vi "Get Computer Resources.vi"(8 "error in (no error)":errorcluster) -> (0 "error out":errorcluster, 3 "Computer Resources":T1)   [LabVIEW 2020]
doc: "This VI collects via the system data API the available computing resources."
uses:
  Type Definitions/Computer Resources.ctl
  Type Definitions/Payload Class.ctl
  Type Definitions/Enum - Metadata.ctl
  <resource>/objmgr/nicontrollersysapi.rc
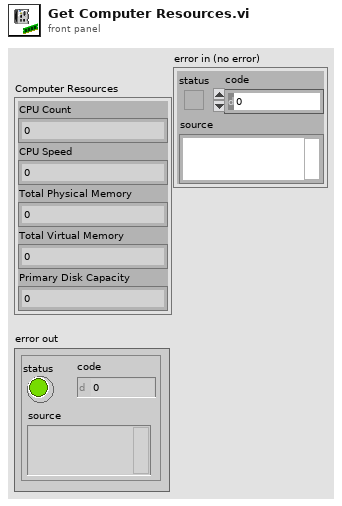
[diagram p1: front panel]
types:
  T1 = typedef "Computer Resources.ctl" = cluster{"CPU Count":i32, "CPU Speed":u32, "Total Physical Memory":dbl, "Total Virtual Memory":dbl, "Primary Disk Capacity":dbl}
  T2 = typedef "Enum - Metadata.ctl" = enum16{"Computer Metadata", "Computer Resources", "RT Image Metadata", "Startup Settings", "Telemetry Recorder Status"}
  T3 = typedef "Payload Class.ctl" = enum16{"System State", "Parameters", "Metadata", "Software Monitor", "Data", "Commands"}
  T4 = typedef "System Resources.ctl" = cluster{"System Session":refnum<k21>, "System Resource":refnum<k20>, "FPGA VI Reference":refnum<k20>}
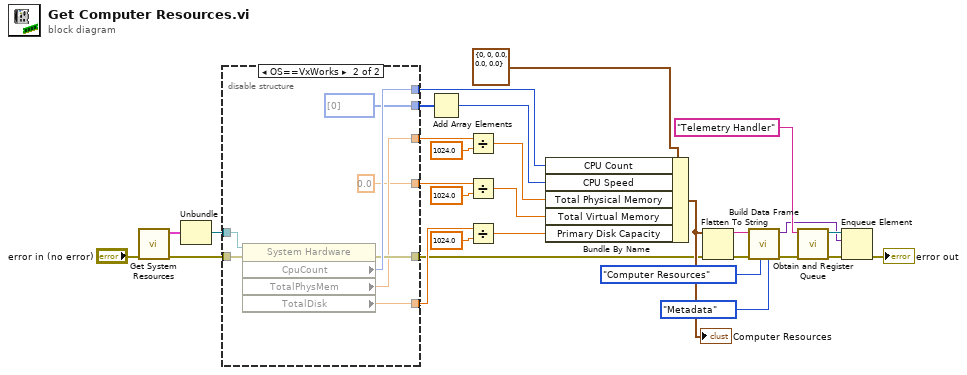
[diagram p0: block diagram]
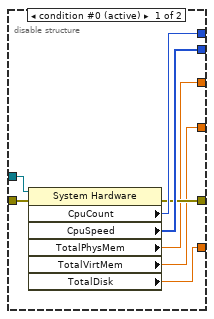
[diagram p2: hidden frame]
diagram:
  n1 = call "Get System Resources.vi"("error in (no error)"="error in (no error)") -> ("error out"=w22:errorcluster, "System Resources"=w25:T4)  [unwired: 9 in]
  n2 = Unbundle(w25) -> ("System Resource"=w24:refnum<k20>)  [unwired: 2 out]
  n3 = disable-structure shown="OS==VxWorks" {
    disable-tunnel: [w37 w45] -> w28
    disable-tunnel: [w36 u32[] [0] ("CpuSpeed")] -> w26
    disable-tunnel: w24 -> [w35 w44]
    disable-tunnel: w22 -> [w34 w43]
    disable-tunnel: [w33 w42] -> w2
    disable-tunnel: [w32 w41] -> w20
    disable-tunnel: [w31 0.0 ("TotalVirtMem")] -> w17
    disable-tunnel: [w30 w40] -> w14
    frame condition #0 (active) {
      n4 = property class="System Hardware"(reference=w35, error in=w34) -> (error out=w33:errorcluster, "CpuCount"=w37:i32, "CpuSpeed"=w36:u32[], "TotalPhysMem"=w30:dbl, "TotalVirtMem"=w31:dbl, "TotalDisk"=w32:dbl)  [unwired: 1 out]
    }
    frame condition #1 {
      n5 = property class="System Hardware"(reference=w44, error in=w43) -> (error out=w42:errorcluster, "CpuCount"=w45:i32, "TotalPhysMem"=w40:dbl, "TotalDisk"=w41:dbl)  [unwired: 1 out]
    }
  }
  n6 = Add Array Elements(numeric array=w26) -> (sum=w29:u32)
  n7 = Divide(x=w14, y=1024.0) -> (x/y=w13:dbl)
  n8 = Divide(x=w17, y=1024.0) -> (x/y=w16:dbl)
  n9 = Divide(x=w20, y=1024.0) -> (x/y=w19:dbl)
  n10 = Bundle By Name(cluster=T1 {"CPU Count"=0, "CPU Speed"=0, "Total Physical Memory"=0.0, "Total Virtual Memory"=0.0, "Primary Disk Capacity"=0.0}, "CPU Count"=w28, "CPU Speed"=w29, "Total Physical Memory"=w13, "Total Virtual Memory"=w16, "Primary Disk Capacity"=w19) -> (w3:T1)
  "Computer Resources" <- w3
  n11 = Flatten To String(anything=w3, error in (no error)=w2) -> (data string=w12:string, error out=w6:errorcluster)  [unwired: 2 in, 1 out]
  n12 = call "Build Data Frame.vi"("Payload Class (Data)"=Payload_Class."Metadata", "Payload ID (0)"=Enum_-_Metadata."Computer Resources" ("Metadata"), "error in (no error)"=w6, "Payload (Empty String)"=w12) -> ("error out"=w5:errorcluster, "Frame"=w4:variant)  [unwired: 6 in]
  n13 = call "Obtain and Register Queue.vi"("error in (no error)"=w5, "name (unnamed)"="Telemetry Handler") -> ("error out"=w9:errorcluster, "Queue Out"=w8:refnum<queue>)  [unwired: 6 in, 2 out]
  n14 = Enqueue Element(queue=w8, element=w4, error in (no error)=w9) -> (error out=→"error out":errorcluster)  [unwired: 1 in, 2 out]
